vi "Show TSUI Error Message.vi"(8 "error in (no error)":errorcluster, 11 "TS Engine Refnum in":refnum<k7>) -> (0 "error out":errorcluster)   [LabVIEW 2015]
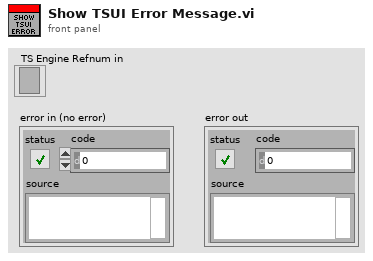
[diagram p1: front panel]
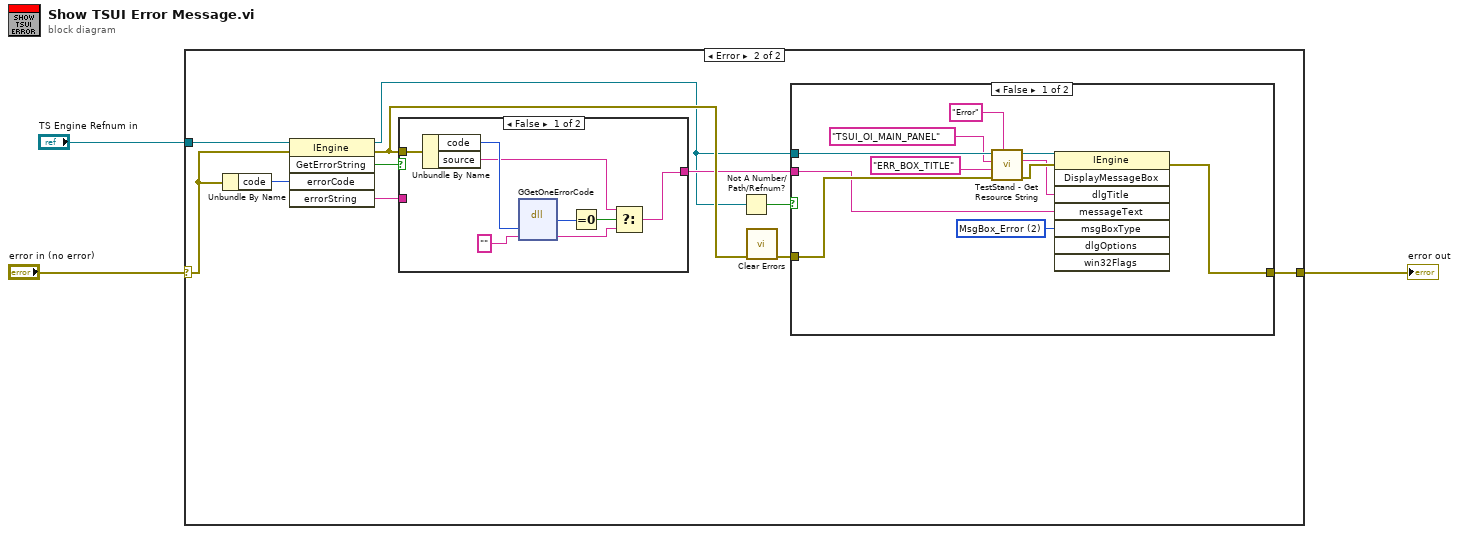
[diagram p0: block diagram]
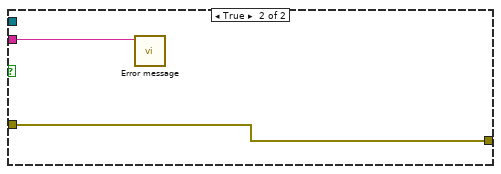
[diagram p3: hidden frame]
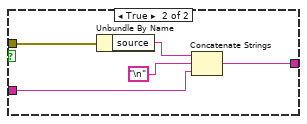
[diagram p4: hidden frame]
diagram:
  n1 = case shown="Error" "error in (no error)" {
    selector: "error in (no error)" -> [w4 w11]
    tunnel: "TS Engine Refnum in" -> [_ w15]
    tunnel: [w4 w5] -> w3
    frame No Error {
    }
    frame Error {
      n2 = Unbundle By Name(w11) -> ("code"=w14:i32)
      n3 = invoke class="IEngine" method="GetErrorString"(reference=w15, error in=w11, "errorCode"=w14) -> (reference out=w6:refnum<k7>, error out=w10:errorcluster, "GetErrorString"=w13:bool, "errorString"=w12:string)  [unwired: 2 in, 1 out]
      n4 = case shown="False" w13 {
        tunnel: w12 -> [_ w38]
        tunnel: w10 -> [w36 w41]
        tunnel: [w29 w37] -> w7
        frame False {
          n5 = Unbundle By Name(w36) -> ("code"=w35:i32, "source"=w31:string)
          n6 = dll-call lib="LabVIEW" fn="GGetOneErrorCode"("errorCode"=w35, "arg2"="") -> ("return type"=w33:u8, "arg2"=w30:string)  [unwired: 4 in, 2 out]
          n7 = Equal To 0?(x=w33) -> (x = 0?=w32:bool)
          n8 = Select(t=w31, s=w32, f=w30) -> (s? t:f=w29:string)
        }
        frame True {
          n9 = Unbundle By Name(w41) -> ("source"=w40:string)
          n10 = Concatenate Strings(w40, "\n", w38) -> (w37:string)
        }
      }
      n11 = Not A Number/Path/Refnum?(number/path/refnum=w6) -> (NaN/Path/Refnum?=w9:bool)
      n12 = call <vilib>:"Clear Errors.vi"("error in (no error)"=w10) -> ("error out"=w8:errorcluster)  [unwired: 5 in, 1 out]
      n13 = case shown="False" w9 {
        tunnel: w8 -> [w23 w28]
        tunnel: [w16 w28] -> w5
        tunnel: w7 -> [w18 w27]
        tunnel: w6 -> [w26 _]
        frame False {
          w17 = 2 items=["MsgBox_Warning", "MsgBox_Information", "MsgBox_Error", "MsgBox_Custom"] ("msgBoxType")
          n14 = call <vilib>:"TestStand - Get Resource String.vi"("Default String"="Error" ("Category"), "error in (no error)"=w23, "Symbol"="ERR_BOX_TITLE", "Category"="TSUI_OI_MAIN_PANEL", "Engine Reference In"=w26) -> ("error out"=w20:errorcluster, "Resource String"=w19:string, "Engine Reference Out"=w21:refnum<k7>)  [unwired: 3 in, 1 out]
          n15 = invoke class="IEngine" method="DisplayMessageBox"(reference=w21, error in=w20, "dlgTitle"=w19, "messageText"=w18, "msgBoxType"=w17) -> (error out=w16:errorcluster)  [unwired: 3 in, 7 out]
        }
        frame True {
          n16 = call "Error message.vi"("Error description"=w27) -> ()  [unwired: 10 in, 1 out]
        }
      }
    }
  }
  "error out" <- w3
